vi "OE1311&OE1351_Query PLL&Overload.vi"(0 "VISA resource name":refnum<visa-resource-name>, 5 "Connection ID in":refnum<k5>, 7 "Timeout":u32=1000, 9 "Remote Mode":u16(ring)=1 items=["RS232"=1, "Ethernet"=3], 11 "Error in (no error)":errorcluster caption="error out（no error）") -> (4 "VISA resource  out":refnum<visa-resource-name>, 6 "Connection ID out":refnum<k5>, 8 "OE1300_Query PLL&Overload":T1, 10 "Output String":string, 15 "Error out":errorcluster caption="error out")   [LabVIEW 2011]
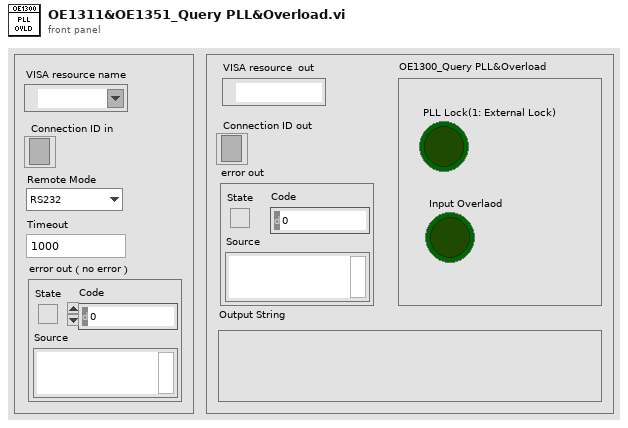
[diagram p1: front panel]
types:
  T1 = cluster{"PLL Lock(1: External Lock)":bool, "Input Overlaod":bool}
  T2 = enum16{"ISRC", "IGND", "ICPL", "ILIN", "PHAS", "FMOD", "RSLP", "FREQ", "SWPT", "SLLM", "SULM", "SSLL", "SSLG", "STLM", "SWRM", "IRNG", "SENS", "RMOD", "OFLT", "OFSL", "SYNC", "DMOD", "HARM", "DARB", "SWVT", "SLVL", "SVLL", "SVUL", "SVSL", "SVSG", "SVTM", "SVRM", "RALL", "SNAP", "OUTP", "OAUX", "COUT", "CAUX", "COFP", "CEXP", "FPOP", "OEXP", "*IDN", "*RST", "OVLD", "INOV", "GNOV", "*PLL", "SSET", "RSET", "AGAN", "APHS", "ARSV", "ASCL", "EQCD", "EQCS", "SPED", "SRAT", "SLEN", "SSLE", "STRG", "SPRM", "STRD", "PAUS", "REST", "SPTS", "TRCA", "TEMP", "RSTU", "IHNZ", "DEQU", "SADD", "ARNG", "CSPE", "ISRCD", "IGNDD", "ICPLD", "ILIND", "PHASD", "FMODD", "RSLPD", "FREQD", "SWPTD", "SLLMD", "SULMD", "SSLLD", "SSLGD", "STLMD", "SWRMD", "SENSD", "RMODD", "OFLTD", "OFSLD", "SYNCD", "HARMD", "EQCDD", "EQCSD", "SNAPD", "OUTPD", "SWVTD", "SLVLD", "SVLLD", "SVULD", "SVSLD", "SVSGD", "SVTMD", "SVRMD", "SVDCD", "ARSVD", "AGAND", "APHSD", "ASCLD", "FPOPD", "CAUXD", "OEXPD", "SPEDD", "SRATD", "SLEND", "SSLED", "STRGD", "SPRMD", "STRDD", "PAUSD", "RESTD", "SPTSD", "TRCAD", "*IDND", "*RSTD", "INOVD", "GNOVD", "*PLLD", "SSETD", "RSETD"}
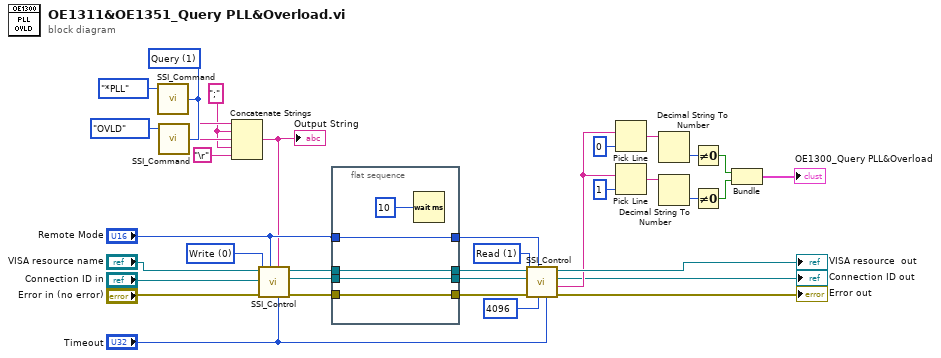
[diagram p0: block diagram]
diagram:
  w11 = ";"
  w22 = u16 1 items=["Write", "Read"] ("Control")
  w15 = u16 1 items=["Set", "Query"] ("Opera")
  w35 = u16 0 items=["Write", "Read"] ("Control")
  n1 = call "SSI_Command.vi"("Opera"=w15, "Command Type"=T2."*PLL") -> ("Output string"=w13:string)  [unwired: 2 in]
  n2 = call "SSI_Command.vi"("Opera"=w15, "Command Type"=T2."OVLD") -> ("Output string"=w12:string)  [unwired: 2 in]
  n3 = Concatenate Strings(w13, w11, w12, w11, "\r") -> (w23:string)
  "Output String" <- w23
  n4 = call "SSI_Control.vi"("Tineout"="Timeout", "Write Buffer"=w23, "Remote Mode"="Remote Mode", "Error in (no error)"="Error in (no error)", "Control"=w35, "Connection ID in"="Connection ID in", "VISA resource name"="VISA resource name") -> ("Error out"=w33:errorcluster, "Connection ID out"=w5:refnum<k5>, "VISA resource  out"=w32:refnum<visa-resource-name>)  [unwired: 1 in, 1 out]
  n5 = flat-sequence {
    tunnel: [w41] -> w31
    tunnel: w33 -> [w41]
    tunnel: [w40] -> w30
    tunnel: w32 -> [w40]
    tunnel: "Remote Mode" -> [w39]
    tunnel: [w39] -> w29
    tunnel: w5 -> [w38]
    tunnel: [w38] -> w4
    frame #0 {
      n6 = Wait (ms)(milliseconds to wait=u32 10 ("等待时间（毫秒）")) -> ()  [unwired: 1 out]
    }
  }
  n7 = call "SSI_Control.vi"("Tineout"="Timeout", "Number of bytes"=u32 4096, "Remote Mode"=w29, "Error in (no error)"=w31, "Control"=w22, "Connection ID in"=w4, "VISA resource name"=w30) -> ("Error out"=→"Error out":errorcluster, "Read Buffer"=w14:string, "Connection ID out"=→"Connection ID out":refnum<k5>, "VISA resource  out"=→"VISA resource  out":refnum<visa-resource-name>)  [unwired: 1 in]
  n8 = Pick Line(multi-line string=w14, line index=0 ("行索引")) -> (output string=w20:string)  [unwired: 1 in]
  n9 = Pick Line(multi-line string=w14, line index=1 ("行索引")) -> (output string=w21:string)  [unwired: 1 in]
  n10 = Decimal String To Number(string=w20) -> (number=w9:i32)  [unwired: 2 in, 1 out]
  n11 = Decimal String To Number(string=w21) -> (number=w10:i32)  [unwired: 2 in, 1 out]
  n12 = Not Equal To 0?(x=w9) -> (x != 0?=w19:bool)
  n13 = Not Equal To 0?(x=w10) -> (x != 0?=w25:bool)
  n14 = Bundle(w19, w25) -> (→"OE1300_Query PLL&Overload":cluster{bool, bool})  [unwired: 1 in]
